vi "applyThreshold.vi"(9 "inIma":sgl[][](array[numeric]), 10 "valSeuil":sgl, 11 "applyThreshold":bool) -> (3 "imaOut":sgl[][](array[numeric]))   [LabVIEW 2020]
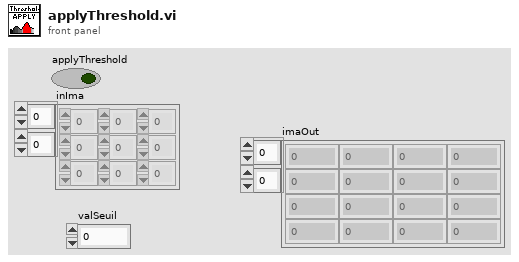
[diagram p1: front panel]
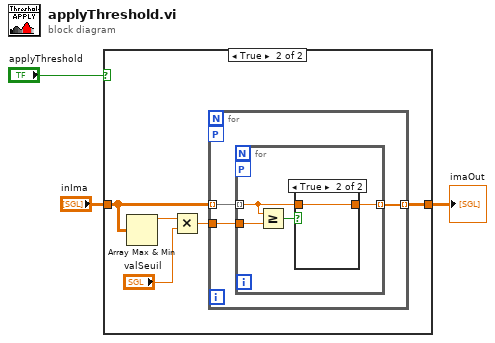
[diagram p0: block diagram]
diagram:
  n1 = case shown="True" "applyThreshold" {
    tunnel: [w4 w6] -> w3
    tunnel: "inIma" -> [w4 w5]
    frame False {
    }
    frame True {
      n2 = Array Max & Min(array=w5) -> (max value=w9:sgl)  [unwired: 3 out]
      n3 = Multiply(x=w9, y="valSeuil") -> (x*y=w7:sgl)
      n4 = for {
        tunnel: w5 -> [w12] mode=indexing
        workers-P: _ -> [_]
        tunnel: w7 -> [w11]
        tunnel: [w10] -> w6 mode=indexing
        n5 = for {
          tunnel: w12 -> [w14] mode=indexing
          workers-P: _ -> [_]
          tunnel: w11 -> [w16]
          tunnel: [w13] -> w10 mode=indexing
          n6 = Greater Or Equal?(x=w14, y=w16) -> (x >= y?=w15:bool)
          n7 = case shown="True" w15 {
            tunnel: [_ w17] -> w13
            tunnel: w14 -> [_ w17]
            frame False {
            }
            frame True {
            }
          }
        }
      }
    }
  }
  "imaOut" <- w3
